vi "Get_reference_samplingdata.vi"(0 "SPU":refnum<k24>, 1 "STSProcess.PDLSTS":refnum<k24>, 2 "Refdata_struct":refnum<k24>[](array[refnum]), 5 "Ref_monitordata_struct":refnum<k24>[](array[refnum]), 7 "MPM":refnum<k24>[](array[refnum]), 9 "SOP":i32, 11 "错误输入（无错误）":errorcluster) -> (6 "PDLSTS out":refnum<k24>, 15 "error out":errorcluster)   [LabVIEW 2017]
doc: "Get logging reference data & add in"
uses:
  D:/test/PDLSTS/LV_PDL_Sample/DLL/STSProcess.dll
  DLL/STSProcess.dll
  D:/test/PDLSTS/LV_PDL_Sample/DLL/InstrumentDLL.dll
  DLL/InstrumentDLL.dll
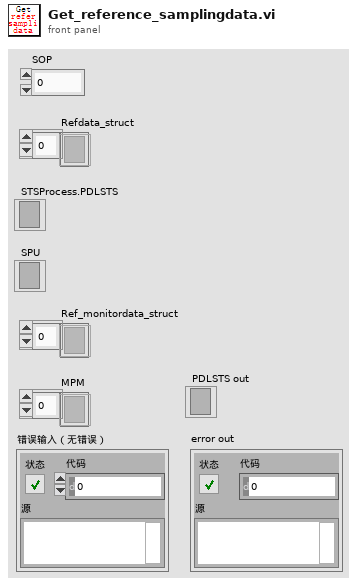
[diagram p1: front panel]
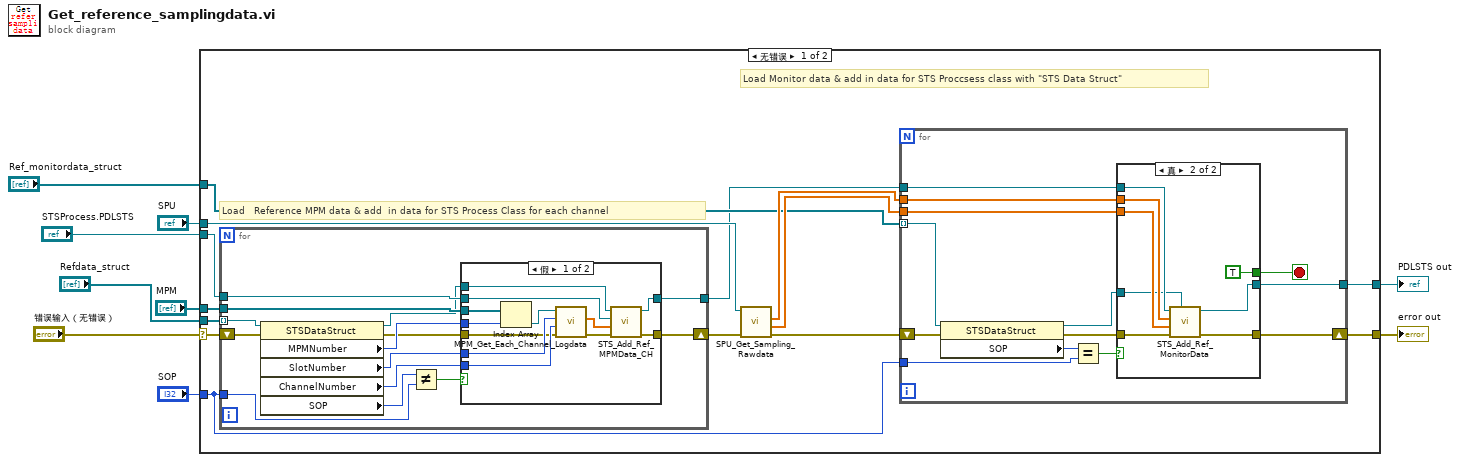
[diagram p0: block diagram]
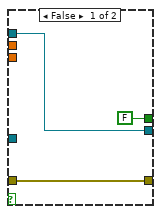
[diagram p2: hidden frame]
diagram:
  n1 = case shown="无错误" "错误输入（无错误）" {
    selector: "错误输入（无错误）" -> [w14 w77]
    tunnel: "STSProcess.PDLSTS" -> [w13 w76]
    tunnel: "Ref_monitordata_struct" -> [w20 _]
    tunnel: "SPU" -> [w19 _]
    tunnel: "MPM" -> [w17 _]
    tunnel: "Refdata_struct" -> [w16 _]
    tunnel: [w15 w77] -> w4
    tunnel: [w11 w76] -> w2
    tunnel: "SOP" -> [w10 _]
    frame No Error {
      # "Load Monitor data & add in data for STS Proccsess class with \"STS Data Struct\""
      # "Load　Reference MPM data & add  in data for STS Process Class for each channel"
      n2 = for {
        tunnel: w16 -> [w56] mode=indexing
        tunnel: w17 -> [w59]
        tunnel: w13 -> [w57]
        shift-right: [w55] -> w18
        shift-left: w14 -> [w53]
        tunnel: [w51] -> w12
        tunnel: w10 -> [w49]
        n3 = property on="属性节点" class="STSDataStruct"(reference=w56, error in=w53) -> (reference out=w52:refnum<k24>, error out=w54:errorcluster, "MPMNumber"=w58:i32, "SlotNumber"=w61:i32, "ChannelNumber"=w60:i32, "SOP"=w50:i32)
        n4 = Not Equal?(x=w50, y=w49) -> (x != y?=w48:bool)
        n5 = case shown="假" w48 {
          tunnel: w61 -> [w73 _]
          tunnel: w60 -> [w72 _]
          tunnel: w59 -> [w71 _]
          tunnel: w58 -> [w70 _]
          tunnel: w57 -> [w69 w75]
          tunnel: [w68 w74] -> w55
          tunnel: w54 -> [w67 w74]
          tunnel: w52 -> [w63 _]
          tunnel: [w62 w75] -> w51
          frame False {
            n6 = Index Array(array=w71, index=w70) -> (element=w66:refnum<k24>)
            n7 = call "MPM_Get_Each_Channel_Logdata.vi"("error in (no error)"=w67, "channelNumber"=w72, "moduleNumber"=w73, ".NET Reference in"=w66) -> ("error out"=w64:errorcluster, "data out"=w65:sgl[])  [unwired: 5 in, 1 out]
            n8 = call "STS_Add_Ref_MPMData_CH.vi"("错误输入（无错误）"=w64, "data"=w65, "STSProcess.PDSTS"=w69, "Setting"=w63) -> ("错误输出"=w68:errorcluster, "PDLSTS"=w62:refnum<k24>)  [unwired: 6 in]
          }
          frame True {
          }
        }
      }
      n9 = call "SPU_Get_Sampling_Rawdata.vi"("错误输入（无错误）"=w18, "SPU"=w19) -> ("error out"=w21:errorcluster, "monitor"=w23:sgl[], "trigger"=w22:sgl[])  [unwired: 5 in, 1 out]
      n10 = for {
        tunnel: w20 -> [w31] mode=indexing
        tunnel: w12 -> [w36]
        tunnel: w22 -> [w35]
        tunnel: w23 -> [w34]
        shift-right: [w33] -> w15
        shift-left: w21 -> [w26]
        tunnel: [w32] -> w11
        tunnel: w10 -> [w29]
        stop <- w24 stop-if-true
        n11 = property class="STSDataStruct"(reference=w31, error in=w26) -> (reference out=w27:refnum<k24>, error out=w25:errorcluster, "SOP"=w30:i32)
        n12 = Equal?(x=w30, y=w29) -> (x = y?=w28:bool)
        n13 = case shown="真" w28 {
          tunnel: w36 -> [w39 w47]
          tunnel: w35 -> [_ w46]
          tunnel: w34 -> [_ w45]
          tunnel: w25 -> [w38 w44]
          tunnel: [w38 w43] -> w33
          tunnel: [w39 w42] -> w32
          tunnel: w27 -> [_ w41]
          tunnel: [FALSE TRUE] -> w24
          frame False {
          }
          frame True {
            n14 = call "STS_Add_Ref_MonitorData.vi"("setting"=w41, "错误输入（无错误）"=w44, "monitorData"=w45, "triggerIndex"=w46, "STSProcess.PDLSTS"=w47) -> ("错误输出"=w43:errorcluster, "PDLSTS out"=w42:refnum<k24>)  [unwired: 5 in]
          }
        }
      }
    }
    frame Error {
    }
  }
  "error out" <- w4
  "PDLSTS out" <- w2
